vi "SetTrigger_SubVI.vi"(7 "ExternalTriggerLevel":dbl, 8 "error in (no error)":errorcluster, 9 "Trigger On":bool, 10 "IVI Refnum in":refnum<k15>, 11 "VISA Refnum in":refnum<visa-resource-name>) -> (0 "error out":errorcluster)   [LabVIEW 2023, in "SpectrumAnalyzerUI.lvlib" / "SpectrumAnalyzerUI.lvclass"]
uses:
  UIs/SpectrumAnalyzerUI/SpectrumAnalyzerUI/SpectrumAnalyzerUI.lvclass
  UIs/SpectrumAnalyzerUI/SpectrumAnalyzerUI/SpectrumAnalyzerUI.lvclass/SpectrumAnalyzerUI.ctl
  <instrlib>/Keysight XSAn/Keysight XSAn.lvlib
  KeysightN9020B.lvlib
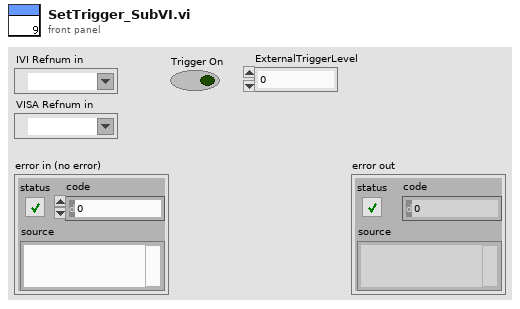
[diagram p1: front panel]
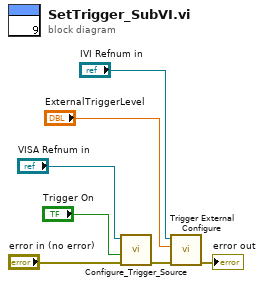
[diagram p0: block diagram]
diagram:
  n1 = call "Configure_Trigger_Source.vi"("error in (no error)"="error in (no error)", "ON/OFF TRIGGER"="Trigger On", "VISA resource name"="VISA Refnum in") -> ("error out"=w1:errorcluster)  [unwired: 7 in, 1 out]
  n2 = call <instrlib>:"Trigger External Configure.vi"("error in (no error)"=w1, "ExternalTriggerLevel"="ExternalTriggerLevel", "instrument handle"="IVI Refnum in") -> ("error out"=→"error out":errorcluster)  [unwired: 7 in, 1 out]
